vi "Request Data JSON.vi"(8 "error in (no error)":errorcluster, 11 "TriggerHotkeyByName in":refnum<class "TriggerHotkeyByName.lvclass">) -> (0 "error out":errorcluster, 2 "Request Data JSON":string, 3 "TriggerHotkeyByName out":refnum<class "TriggerHotkeyByName.lvclass">)   [LabVIEW 2022 SP3, in "obs-websocket-lv.lvlib" / "TriggerHotkeyByName.lvclass"]
uses:
  TriggerHotkeyByName.lvclass
  TriggerHotkeyByName.lvclass/TriggerHotkeyByName.ctl
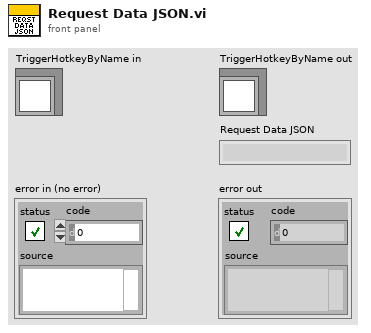
[diagram p1: front panel]
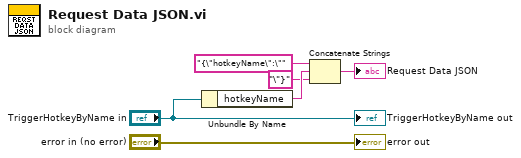
[diagram p0: block diagram]
diagram:
  n1 = Unbundle By Name("TriggerHotkeyByName in") -> ("hotkeyName"=w3:string)
  n2 = Concatenate Strings("{\"hotkeyName\":\"", w3, "\"}") -> (→"Request Data JSON":string)
  "error out" <- "error in (no error)"
  "TriggerHotkeyByName out" <- "TriggerHotkeyByName in"
